vi "LabVIEW Basics #10 - Servo Control.vi"() -> ()   [LabVIEW 2020]
uses:
  <vilib>/MakerHub/LINX/Public/Utilities/Open Serial.vi
  <vilib>/MakerHub/LINX/Public/Sensors/Motion/Servo/Servo Open N Channels.vi
  <vilib>/MakerHub/LINX/Public/Sensors/Motion/Servo/Servo Set Pulse Width N Channels.vi
  <vilib>/MakerHub/LINX/Public/Sensors/Motion/Servo/Servo Close N Channels.vi
  <vilib>/MakerHub/LINX/LMH-LINX.lvlib
  <vilib>/MakerHub/LINX/Public/Sensors/Motion/Servo/Servo.lvlib
panel:
  in  "Tilt Servo":u16(slide) step=100 scale=500.0..2500.0
  in  "Pan Servo":u16(slide) step=100 scale=500.0..2500.0
  in  "Servo Channels":u8[](array[numeric])
  out "Device Name":string
  in  "Stop":bool
  # "General Controls"
  # "Servo Controls"
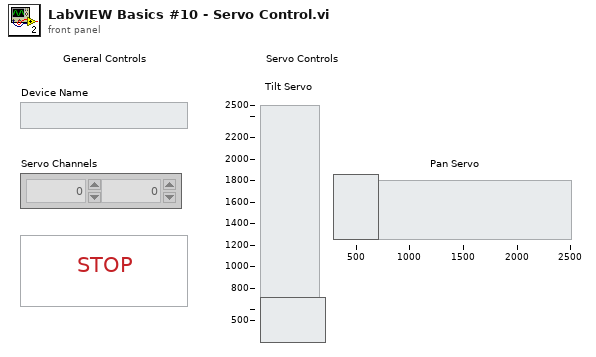
[diagram p1: front panel]
types:
  T1 = typedef "LMH-LINX.lvlib/LINX Ref.ctl" = cluster{"IO":T2, "Interface":T3, "LINX Device Config":T4}
  T2 = typedef "LMH-LINX.lvlib/Platform.ctl" = enum16{"Remote", "Local"}
  T3 = typedef "LMH-LINX.lvlib/Interface.ctl" = enum16{"Serial", "TCP"}
  T4 = typedef "LMH-LINX.lvlib/Device.lvlib/LINX Device Config.ctl" = cluster{"Interface":T3, "COM Port":refnum<visa-resource-name>, "TCP Configuration":T5, "Device Family":u8, "Device ID":u8, "Device Name":string, "TCP Ref":refnum<k5>, "Channels":T6}
  T5 = typedef "LMH-LINX.lvlib/Device.lvlib/TCP Config.ctl" = cluster{"IP Address":string, "Port":u16}
  T6 = typedef "LMH-LINX.lvlib/Channels.ctl" = cluster{"DI":u8[], "DO":u8[], "AI":u8[], "AO":u8[], "PWM":u8[], "QE":u8[], "UART":u8[], "I2C 2":u8[], "SPI":u8[], "CAN":u8[], "Servo":u8[], "AI Ref (V)":dbl, "AI Resolution (Bits)":u8, "AO Ref (V)":dbl, "AO Resolution (Bits)":u8}
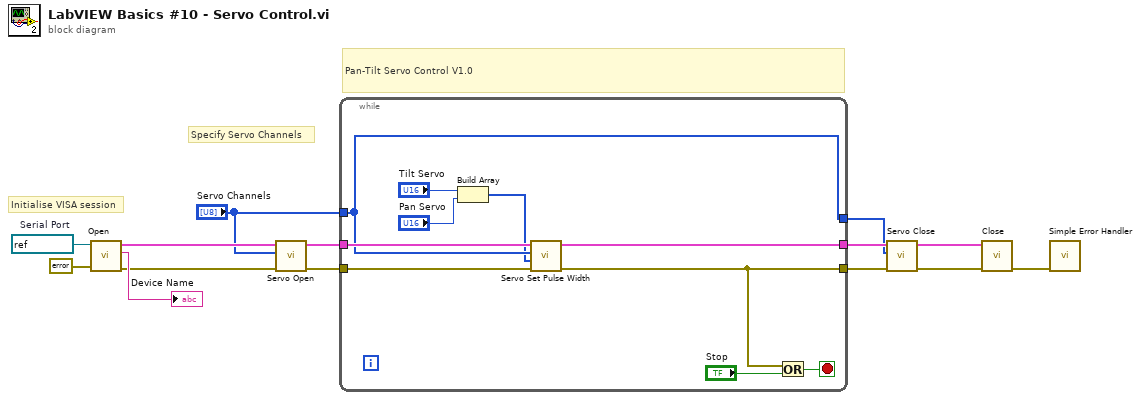
[diagram p0: block diagram]
diagram:
  w14 = refnum<visa-resource-name> "COM5"  # Serial Port
  # "Specify Servo Channels"
  # "Initialise VISA session"
  # "Pan-Tilt Servo Control V1.0"
  n1 = call-poly <vilib>:"Open.vi"("Error In"=errorcluster {"status"=FALSE, "code"=0, "source"=""}, "Serial Port"=w14) -> ("Error Out"=w7:errorcluster, "Device Name"=→"Device Name":string, "LINX Resource"=w6:T1)  [unwired: 7 in]
  n2 = call-poly <vilib>:"Servo Open.vi"("Error In"=w7, "Servo Channels"="Servo Channels", "LINX Resource"=w6) -> ("Error Out"=w5:errorcluster, "LINX Resource"=w8:T1)  [unwired: 7 in]
  n3 = while {
    tunnel: w8 -> [w22]
    tunnel: w5 -> [w21]
    tunnel: [w19] -> w4
    tunnel: [w20] -> w3
    tunnel: "Servo Channels" -> [w18]
    tunnel: [w18] -> w1
    stop <- w23 stop-if-true
    n4 = Build Array("Tilt Servo", "Pan Servo") -> (w17:u16[])
    n5 = call-poly <vilib>:"Servo Set Pulse Width.vi"("Error In"=w21, "Pulse Widths (uS)"=w17, "Servo Channels"=w18, "LINX Resource"=w22) -> ("Error Out"=w19:errorcluster, "LINX Resource"=w20:T1)  [unwired: 6 in]
    n6 = Or(x=w19, y="Stop") -> (x .or. y?=w23:bool)
  }
  n7 = call-poly <vilib>:"Servo Close.vi"("Error In"=w4, "Servo Channels"=w1, "LINX Resource"=w3) -> ("Error Out"=w10:errorcluster, "LINX Resource"=w9:T1)  [unwired: 7 in]
  n8 = call <vilib>:"Close.vi"("Error In"=w10, "LINX Resource"=w9) -> ("Error Out"=w11:errorcluster)  [unwired: 9 in]
  n9 = call <vilib>:"Simple Error Handler.vi"("error in (no error)"=w11) -> ()  [unwired: 4 in, 5 out]
